vi "FPGA_VI_III.vi"() -> ()   [LabVIEW 2017]
uses:
  <vilib>/rvi/Emulation/niFpgaGetClockAttributes.vi
  <vilib>/rvi/Emulation/niFpgaSctlEmulationGetInTimedLoop.vi
  <vilib>/rvi/Emulation/niFpgaEmulationReportErrorSimple.vi
  <vilib>/rvi/DataTransferAndStorage/Container/Common/niFpgaContainerGetUniqueNameForEmu.vi
  <vilib>/rvi/DataTransferAndStorage/Container/Common/niFpgaContainerSetEmuInfo.vi
  <vilib>/rvi/eio/common/nirviEmuReportErrorAndStop.vi
  <vilib>/rvi/DataTransferAndStorage/Container/Common/niFpgaContainerExecOnDevCompGetState.vi
  <vilib>/rvi/Emulation/niFpgaEmulationIsFPGAContextNoSignature.vi
  <vilib>/rvi/errors/niFpgaSetErrorForExecOnDevCompSimple.vi
  <vilib>/rvi/FIFO/Fifo_Resource/nirvififoEmulationSetSize.vi
  <vilib>/rvi/FIFO/Fifo_Resource/nirviFifoEmulationQueueMgr.vi
  <instcachedir>/0/nirviFifoEmulationQueueMgr_E5CAEC123FF24DC58D834DCA3CDAA9B5.lvgen/nirviFifoEmulationQueueMgr_E5CAEC123FF24DC58D834DCA3CDAA9B5_003.vi
  <vilib>/rvi/FIFO/Fifo_Resource/nirvififoEmulationDetermineInputValidOut.vi
  <vilib>/rvi/FIFO/Fifo_Resource/nirvififoEmulationCreateLock.vi
  <vilib>/rvi/Emulation/niFpgaProcessEmulError.vi
  <vilib>/rvi/FIFO/Fifo_Resource/nirvififoEmulationObtainLock.vi
  <vilib>/rvi/FIFO/Fifo_Resource/nirvififoEmulationReleaseLock.vi
  <vilib>/rvi/occurrence/nirviWaitOnOccurrenceBase.vi
  <vilib>/rvi/errors/nirviReportUnexpectedCaseInternalError.vi
  <vilib>/rvi/errors/nirviReportUnexpectedCaseInternalError (U32).vi
  <vilib>/Utility/error.llb/Clear Errors.vi
  <vilib>/rvi/interface/RandomDataEmulation/niFpgaRandomDataHandleErrors.vi
  <vilib>/rvi/Emulation/niFpgaCriticalErrorInLSC.vi
  <vilib>/rvi/eio/common/nirviEmuTemplateMethod_errors.vi
  <vilib>/rvi/LocalResourceManager/LocalResourceManager.xnode
  <vilib>/rvi/DataTransferAndStorage/Container/XNode/niFpgaContainer.xnode
  <vilib>/rvi/FIFO/Fifo_Resource/niFpgaFifoEmulationRefIn.vi
  <vilib>/eio/EIONode/EIONode.xnode
panel:
  out "Mod3/DIO1":bool
  out "s? t:f":bool
  out "Element":bool
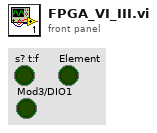
[diagram p1: front panel]
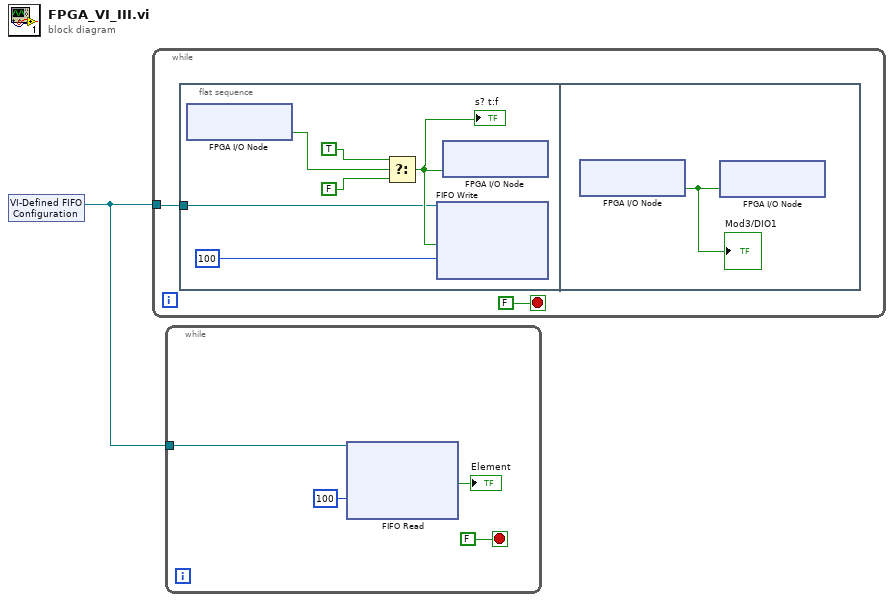
[diagram p0: block diagram]
diagram:
  n1 = xnode "VI-Defined FIFO Configuration"() -> ("FIFO Out"=w1:refnum<k21>)
  n2 = while {
    tunnel: w1 -> [w2]
    stop <- FALSE stop-if-true
    n3 = flat-sequence {
      tunnel: w2 -> [w5]
      frame #0 {
        n4 = xnode "FPGA I/O Node"() -> ("Mod3/DIO0"=w4:bool)  [unwired: 1 in, 1 out]
        n5 = Select(t=TRUE, s=w4, f=FALSE) -> (s? t:f=w7:bool)
        "s? t:f" <- w7
        n6 = xnode ("FIFO Write")("Element"=w7, "Timeout"=100, "FIFO In"=w5) -> ()  [unwired: 2 out]
        n7 = xnode "FPGA I/O Node"("Mod3/DIO1"=w7) -> ()  [unwired: 1 in, 1 out]
      }
      frame #1 {
        n8 = xnode "FPGA I/O Node"() -> ("Mod3/DIO1"=w10:bool)  [unwired: 1 in, 1 out]
        "Mod3/DIO1" <- w10
        n9 = xnode "FPGA I/O Node"("Mod3/DIO2"=w10) -> ()  [unwired: 1 in, 1 out]
      }
    }
  }
  n10 = while {
    tunnel: w1 -> [w13]
    stop <- FALSE stop-if-true
    n11 = xnode ("FIFO Read")("Timeout"=100, "FIFO In"=w13) -> ("Element"=→"Element":bool)  [unwired: 2 out]
  }
